vi "Read New.vi"(8 "Error In":errorcluster, 11 "Set Delimiter In":refnum<class "SetDelimiter.lvclass">) -> (0 "Error Out":errorcluster, 2 "New Value":cluster{"Close":string, "Open":string}, 3 "Set Delimiter Out":refnum<class "SetDelimiter.lvclass">)   [LabVIEW 2018, in "Toolkit.lvlib" / "Tokens.lvlib" / "SetDelimiter.lvclass"]
doc: "Gets the new opening and closing components of the delimiter.\n\n<B>Set Delimiter In/Out</B> - Represents a Set Delimiter token in a lexed Mustache template.\n\n<B>New Value</B> - The open and close components that delimit, or surround, the next Mustache tags."
uses:
  SetDelimiter.lvclass
  SetDelimiter.lvclass/SetDelimiter.ctl
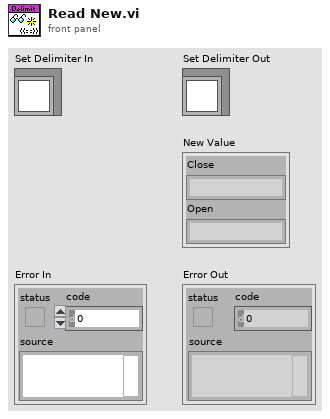
[diagram p1: front panel]
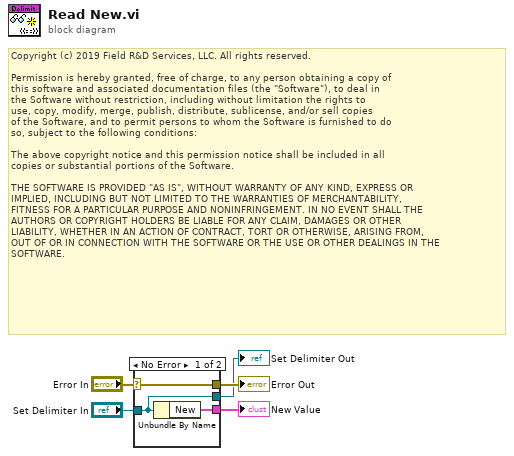
[diagram p0: block diagram]
diagram:
  # "Copyright (c) 2019 Field R&D Services, LLC. All rights reserved.\n\nPermission is hereby granted, free of charge, to any person obtaining a copy of\nthis software and associated documentation files (the \"Software\"), to deal in\nthe Software without restriction, including without limitation the rights to\nuse, copy, modify, merge, publish, distribute, sublicense, and/or sell copies\nof the Software, and to permit persons to whom the Software is furnished to do\nso, subject to the following conditions:\n\nThe above copyright notice and this permission notice shall be included in all\ncopies or substantial portions of the Software.\n\nTHE SOFTWARE IS PROVIDED \"AS IS\", WITHOUT WARRANTY OF ANY KIND, EXPRESS OR\nIMPLIED, INCLUDING BUT NOT LIMITED TO THE WARRANTIES OF MERCHANTABILITY,\nFITNESS FOR A PARTICULAR PURPOSE AND NONINFRINGEMENT. IN NO EVENT SHALL THE\nAUTHORS OR COPYRIGHT HOLDERS BE LIABLE FOR ANY CLAIM, DAMAGES OR OTHER\nLIABILITY, WHETHER IN AN ACTION OF CONTRACT, TORT OR OTHERWISE, ARISING FROM,\nOUT OF OR IN CONNECTION WITH THE SOFTWARE OR THE USE OR OTHER DEALINGS IN THE\nSOFTWARE."
  n1 = case shown="No Error" "Error In" {
    selector: "Error In" -> [w8 w9]
    tunnel: [w8 w9] -> w4
    tunnel: [w7 w10] -> w2
    tunnel: "Set Delimiter In" -> [w7 w10]
    tunnel: [w6 _] -> w1
    frame No Error {
      n2 = Unbundle By Name(w7) -> ("New"=w6:cluster{"Close":string, "Open":string})
    }
    frame Error {
    }
  }
  "Error Out" <- w4
  "Set Delimiter Out" <- w2
  "New Value" <- w1
